vi "Init String.vi"(8 "error in (no error)":errorcluster, 10 "String":string) -> (0 "error out":errorcluster, 3 "StringStream out":refnum<class "StringStream.lvclass">)   [LabVIEW 2020, in "IO.lvlib" / "StringStream.lvclass"]
uses:
  StringStream.lvclass
  StringStream.lvclass/StringStream.ctl
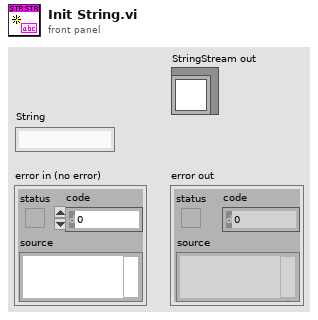
[diagram p1: front panel]
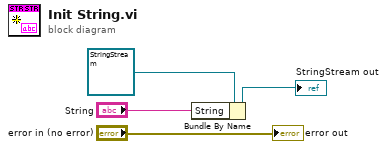
[diagram p0: block diagram]
diagram:
  n1 = Bundle By Name(cluster=refnum<class "StringStream.lvclass"> refnum ("StringStream in"), "String"="String") -> (→"StringStream out":refnum<class "StringStream.lvclass">)
  "error out" <- "error in (no error)"
